vi "actuatorLimits.vi"(8 "valorMinimo":dbl, 9 "valorMaximo":dbl, 10 "valorEntrada":dbl) -> (2 "valorSalida":dbl, 3 "fueraDelEspacioDeTrabajo":bool)   [LabVIEW 2019]
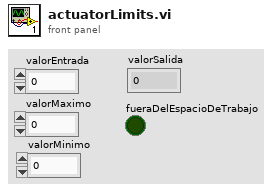
[diagram p1: front panel]
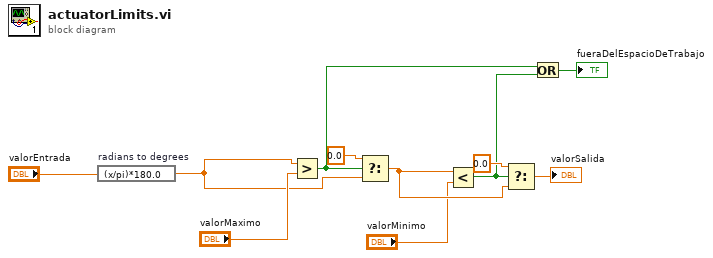
[diagram p0: block diagram]
diagram:
  n1 = expression code="(x/pi)*180.0" "radians to degrees"("valorEntrada") -> (w5:dbl)
  n2 = Greater?(x=w5, y="valorMaximo") -> (0:w2:bool)
  n3 = Select(t=0.0, s=w2, f=w5) -> (s? t:f=w9:dbl)
  n4 = Less?(x=w9, y="valorMinimo") -> (x < y?=w3:bool)
  n5 = Select(t=0.0, s=w3, f=w9) -> (s? t:f=→"valorSalida":dbl)
  n6 = Or(x=w2, y=w3) -> (x .or. y?=→"fueraDelEspacioDeTrabajo":bool)
